vi "CaseStructure - Case Name to Group Name.vi"(11 "element":string) -> (3 "String":string)   [LabVIEW 2017, in "csmHelper-CaseStructure.lvlib"]
doc: "-- <b>输入控件</b> --\n- <b>element</b>:\n\n\n-- <b>输出控件</b> --\n- <b>String</b>:"
uses:
  csmHelper-CaseStructure.lvlib
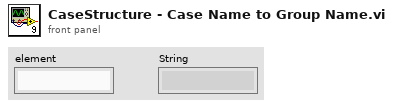
[diagram p1: front panel]
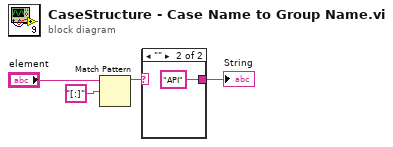
[diagram p0: block diagram]
diagram:
  n1 = Match Pattern(string="element", regular expression="[:]") -> (before substring=w1:string)  [unwired: 1 in, 3 out]
  n2 = case shown="\"\"" w1 {
    selector: w1 -> [w5 _]
    tunnel: [w5 "API"] -> w3
    frame "False", Default {
    }
    frame "" {
    }
  }
  "String" <- w3
